vi "Renishaw-XL80_GetCancelPreHeat.vi"(8 "error in (no error)":errorcluster, 11 "Renishaw-XL80 in":refnum<class "Renishaw-XL80.lvclass">) -> (0 "error out":errorcluster, 3 "Renishaw-XL80 out":refnum<class "Renishaw-XL80.lvclass">)   [LabVIEW 2024, in "Renishaw-XL80.lvclass"]
uses:
  Renishaw-XL80.lvclass
  Renishaw-XL80.lvclass/Renishaw-XL80.ctl
  D:/A.C.M/Example CSharp_64/bin/Debug/Interop.DX10SDKADAPTORLib.dll
  Example CSharp_64/bin/Debug/Interop.DX10SDKADAPTORLib.dll
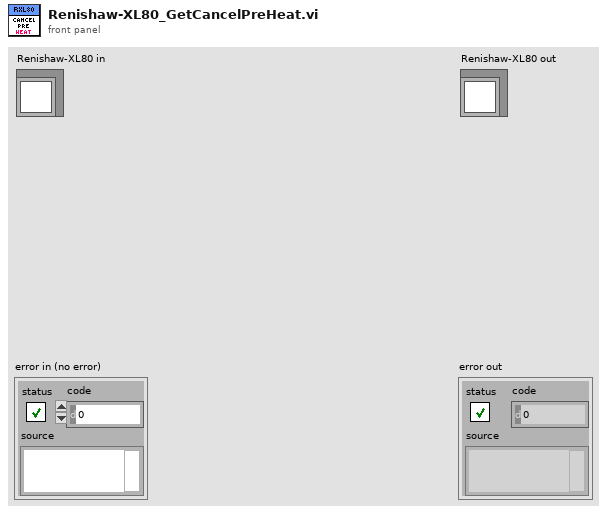
[diagram p1: front panel]
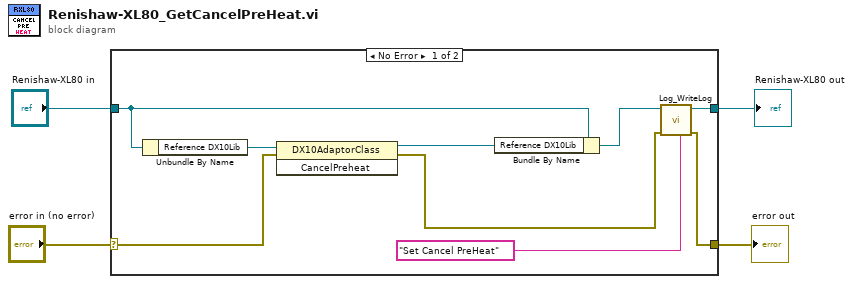
[diagram p0: block diagram]
diagram:
  n1 = case shown="No Error" "error in (no error)" {
    selector: "error in (no error)" -> [w11 w15]
    tunnel: [w7 w15] -> w1
    tunnel: [w8 w14] -> w2
    tunnel: "Renishaw-XL80 in" -> [w10 w14]
    frame No Error {
      n2 = Unbundle By Name(w10) -> ("Reference DX10Lib"=w13:refnum<k24>)
      n3 = invoke class="DX10AdaptorClass" method="CancelPreheat"(reference=w13, error in=w11) -> (reference out=w12:refnum<k24>, error out=w5:errorcluster)  [unwired: 1 in, 1 out]
      n4 = Bundle By Name(cluster=w10, "Reference DX10Lib"=w12) -> (w9:refnum<class "Renishaw-XL80.lvclass">)
      n5 = call-dynamic "Log_WriteLog.vi"("Additional text"="Set Cancel PreHeat", "error in (no error)"=w5, "Log in"=w9) -> ("error out"=w7:errorcluster, "Log out"=w8:refnum<class "Renishaw-XL80.lvclass">)  [unwired: 7 in]
    }
    frame Error {
    }
  }
  "error out" <- w1
  "Renishaw-XL80 out" <- w2
